vi "Operate Relay.vi"(8 "error in (no error)":errorcluster, 10 "Relay (ON)":bool=TRUE, 11 "VISA resource name":refnum<visa-resource-name>) -> (0 "error out":errorcluster, 3 "VISA resource name out":refnum<visa-resource-name>)   [LabVIEW 2013, in "Watts Up PRO Net Series.lvlib"]
doc: "Changes the state of the relay switch. Useful for programatically powering off devices.\n\n<b>Note:</b> Relay switch is only available on Watts Up .Net models."
uses:
  <instrlib>/Watts Up PRO Net Series/Watts Up PRO Net Series.lvlib
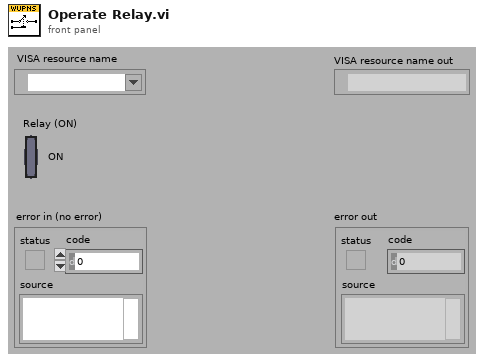
[diagram p1: front panel]
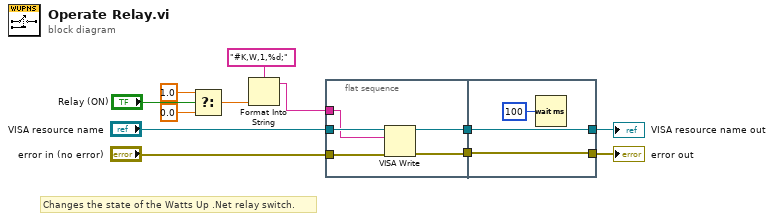
[diagram p0: block diagram]
diagram:
  # "Changes the state of the Watts Up .Net relay switch."
  n1 = Select(t=1.0, s="Relay (ON)", f=0.0) -> (s? t:f=w3:dbl)
  n2 = Format Into String(format string="#K,W,1,%d;", w3) -> (resulting string=w1:string)  [unwired: 2 in, 1 out]
  n3 = flat-sequence {
    tunnel: "VISA resource name" -> [w17]
    tunnel: "error in (no error)" -> [w16]
    tunnel: [w15] -> w8
    tunnel: [w14] -> w7
    tunnel: w1 -> [w13]
    tunnel: [w19] -> w9
    tunnel: [w20] -> w10
    tunnel: w8 -> [w20]
    tunnel: w7 -> [w19]
    frame #0 {
      n4 = VISA Write(VISA resource name=w17, write buffer=w13, error in (no error)=w16) -> (VISA resource name out=w15:refnum<visa-resource-name>, error out=w14:errorcluster)  [unwired: 1 out]
    }
    frame #1 {
      n5 = Wait (ms)(milliseconds to wait=u32 100) -> ()  [unwired: 1 out]
    }
  }
  "VISA resource name out" <- w10
  "error out" <- w9
